vi "Load Factor.vi"(8 "error in":errorcluster, 11 "Parrot in":refnum<class "Parrot.lvclass">) -> (0 "error out":errorcluster, 2 "Load Factor":dbl, 3 "Parrot out":refnum<class "Parrot.lvclass">)   [LabVIEW 2020, in "Parrot.lvclass"]
uses:
  Parrot.lvclass
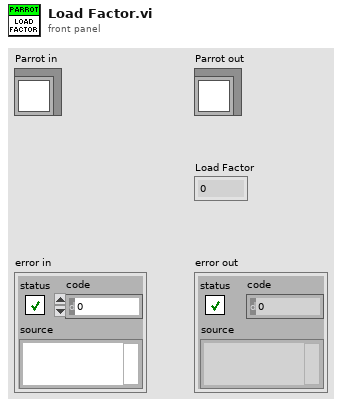
[diagram p1: front panel]
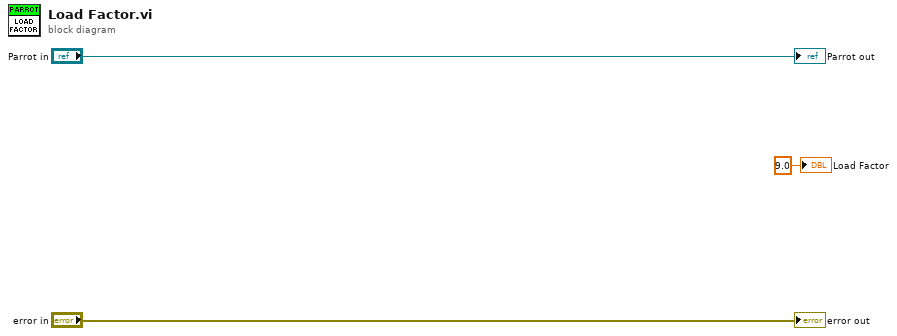
[diagram p0: block diagram]
diagram:
  "error out" <- "error in"
  "Parrot out" <- "Parrot in"
  "Load Factor" <- 9.0 ("Load Factor")
